vi "EventRobotResponding.vi"(9 "IA State 2":T1) -> (1 "Robot responding status":dbl[](array[numeric]), 2 "Is there a robot not responding?":bool)   [LabVIEW 2016]
uses:
  Core/AI Input.ctl
  Core/AI Robot.ctl
  Intel/Functions Enum.ctl
  Intel/AttackerStates.ctl
  Core/AI Ball.ctl
  Core/Field Size.ctl
  Core/AI Judge.ctl
  Intel/Command Enum.ctl
  Events.ctl
panel:
  in  "Array 2":bool[](array[boolean])
  in  "Array":dbl[](array[numeric])=[1.0, 1.0, 1.0, 1.0, 1.0, 1.0]
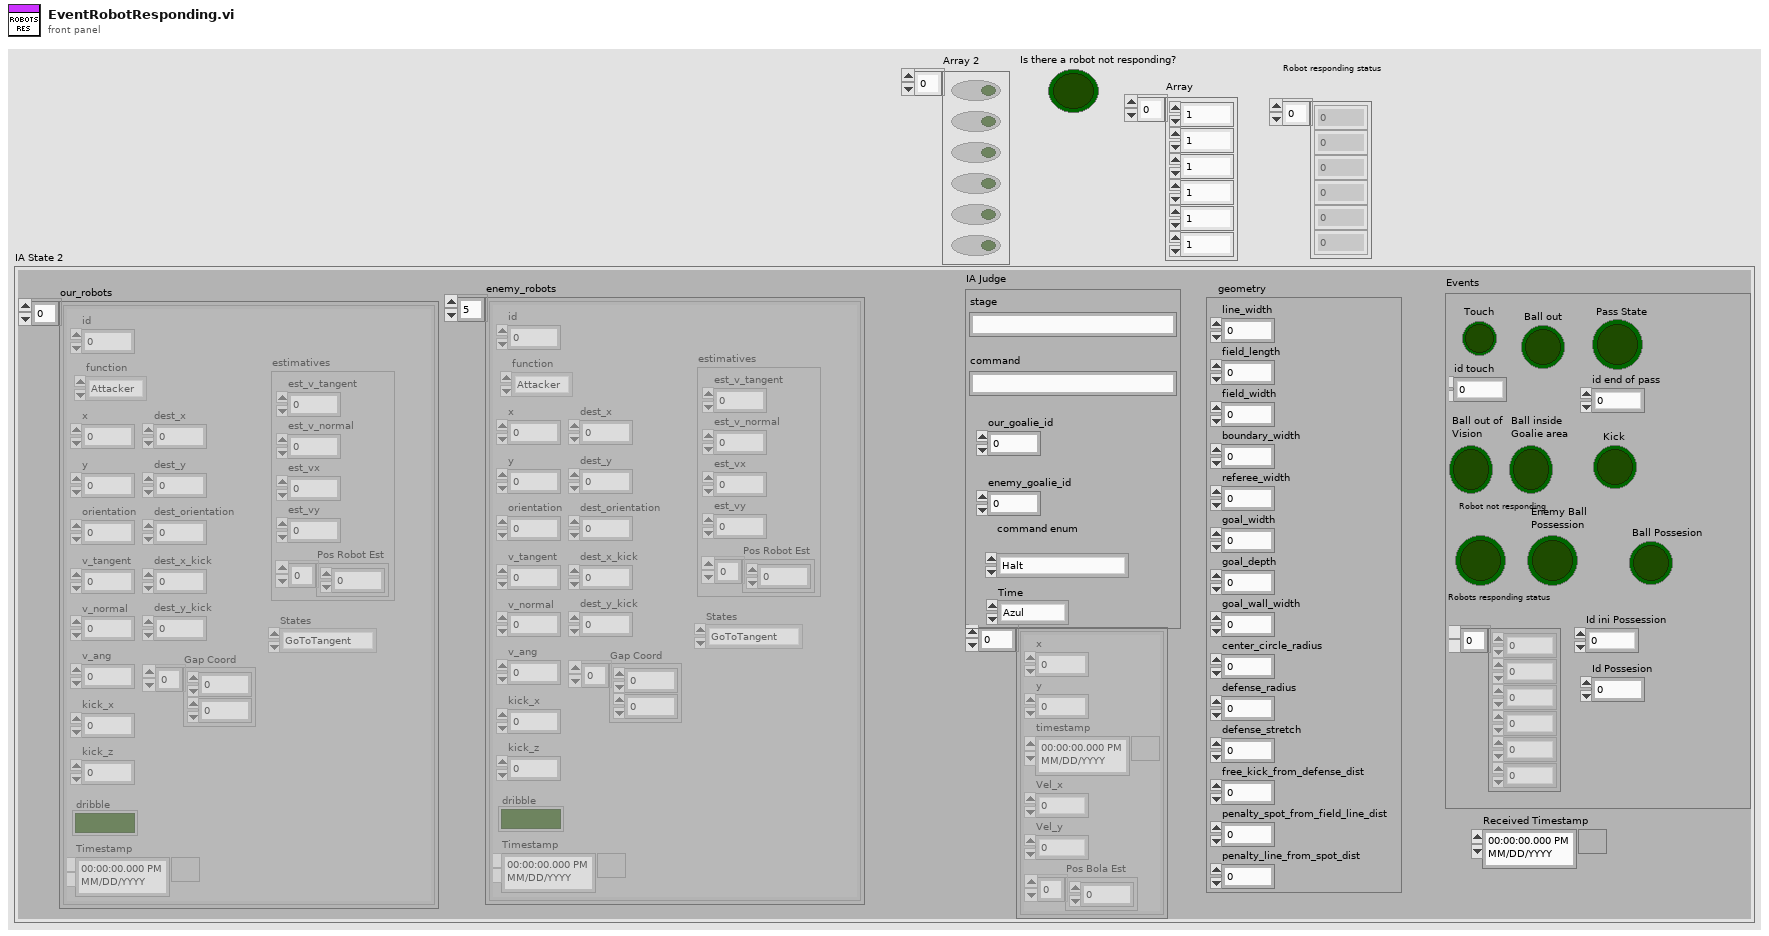
[diagram p1: front panel]
types:
  T1 = typedef "AI Input.ctl" = cluster{"our_robots":T2[], "enemy_robots":T2[], "balls":T5[], "geometry":T6, "IA Judge":T7, "Received Timestamp":timestamp, "Events":T9}
  T2 = typedef "AI Robot.ctl" = cluster{"id":u32, "function":T3, "x":dbl, "y":dbl, "orientation":dbl, "v_tangent":dbl, "v_normal":dbl, "v_ang":dbl, "kick_x":dbl, "kick_z":dbl, "dribble":bool, "Timestamp":timestamp, "dest_x":dbl, "dest_y":dbl, "dest_orientation":dbl, "estimatives":cluster{"est_v_tangent":dbl, "est_v_normal":dbl, "est_vx":dbl, "est_vy":dbl, "Pos Robot Est":dbl[]}, "dest_x_kick":dbl, "dest_y_kick":dbl, "Gap Coord":dbl[], "States":T4}
  T3 = typedef "Functions Enum.ctl" = enum16{"Attacker", "Goalie", "Defender", "Striker", "Goto 0", "Dummy", "Kicker", "ZigZag"}
  T4 = typedef "AttackerStates.ctl" = enum16{"Pass", "GoToTangent", "BallGetting", "GoToKick", ""}
  T5 = typedef "AI Ball.ctl" = cluster{"x":dbl, "y":dbl, "timestamp":timestamp, "Vel_x":dbl, "Vel_y":dbl, "Pos Bola Est":dbl[]}
  T6 = typedef "Field Size.ctl" = cluster{"line_width":u32, "field_length":u32, "field_width":u32, "boundary_width":u32, "referee_width":u32, "goal_width":u32, "goal_depth":u32, "goal_wall_width":u32, "center_circle_radius":u32, "defense_radius":u32, "defense_stretch":u32, "free_kick_from_defense_dist":u32, "penalty_spot_from_field_line_dist":u32, "penalty_line_from_spot_dist":u32}
  T7 = typedef "AI Judge.ctl" = cluster{"stage":string, "command":string, "our_goalie_id":dbl, "enemy_goalie_id":dbl, "command enum":T8, "Time":enum16{"Azul", "Amarelo"}}
  T8 = typedef "Command Enum.ctl" = enum16{"Halt", "Stop", "Force Start", "PKA Normal Start", "Prepare Kickoff Ally", "PKE Normal Start", "Prepare Kickoff Enemy", "Prepare Penalty Ally", "PPA Normal Start", "Prepare Penalty Enemy", "PPE Normal Start", "Direct Free Enemy", "Direct Free Ally", "Indirect Free Enemy", "Indirect Free Ally", "Timeout Enemy", "Timeout Ally", "Goal Enemy", "Goal Ally", "Ball Placement Enemy", "Ball Placement Ally", "Normal Half Time", "Extra Time Break", "Extra Half Time", "None", "Post Game"}
  T9 = typedef "Events.ctl" = cluster{"Touch":bool, "Ball out":bool, "id touch":dbl, "Ball out of \nVision":bool, "Ball inside \nGoalie area":bool, "Robot not responding":bool, "Robots responding status":dbl[], "Enemy Ball \nPossession":bool, "Pass State":bool, "id end of pass":dbl, "Kick":bool, "Id ini Possession":dbl, "Ball Possesion":bool, "Id Possesion":dbl}
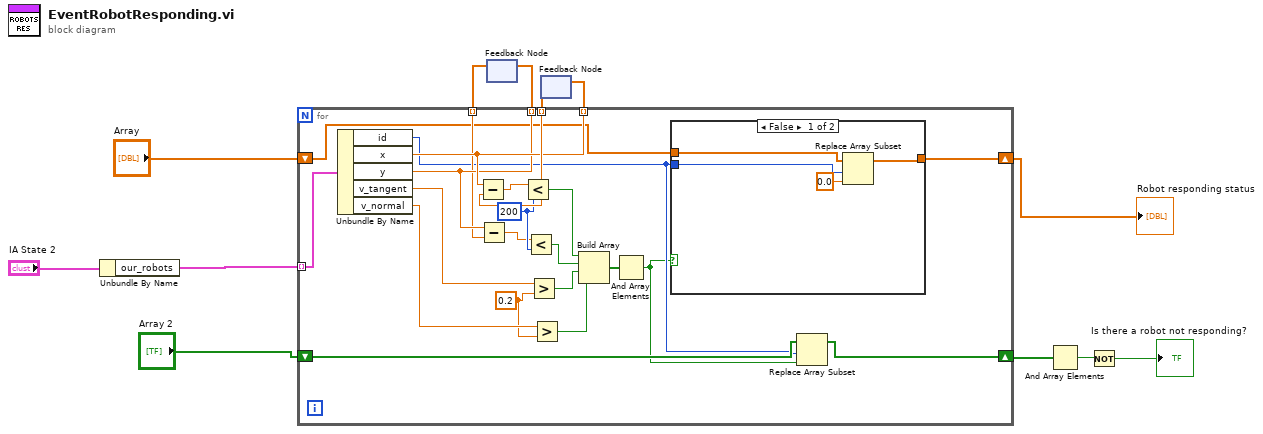
[diagram p0: block diagram]
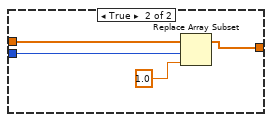
[diagram p2: hidden frame]
diagram:
  n1 = Unbundle By Name("IA State 2") -> ("our_robots"=w11:T2[])
  n2 = feedback #1() -> (w7:dbl[])  [unwired: 1 in]
  n3 = feedback #2() -> (w8:dbl[])  [unwired: 1 in]
  n4 = for {
    tunnel: w11 -> [w34] mode=indexing
    tunnel: [w32] -> w10 mode=indexing
    tunnel: [w31] -> w9 mode=indexing
    tunnel: w8 -> [w33] mode=indexing
    tunnel: w7 -> [w30] mode=indexing
    shift-right: [w18] -> w5
    shift-left: "Array" -> [w17]
    shift-right: [w13] -> w3
    shift-left: "Array 2" -> [w16]
    w24 = 0.2 ("y")
    w28 = 200
    n5 = Unbundle By Name(w34) -> ("id"=w15:u32, "x"=w32:dbl, "y"=w31:dbl, "v_tangent"=w26:dbl, "v_normal"=w25:dbl)
    n6 = Subtract(x=w32, y=w33) -> (x-y=w29:dbl)
    n7 = Subtract(x=w31, y=w30) -> (x-y=w27:dbl)
    n8 = Less?(x=w29, y=w28) -> (x < y?=w23:bool)
    n9 = Less?(x=w27, y=w28) -> (x < y?=w22:bool)
    n10 = Greater?(x=w26, y=w24) -> (0:w21:bool)
    n11 = Greater?(x=w25, y=w24) -> (0:w20:bool)
    n12 = Build Array(w23, w22, w21, w20) -> (w19:bool[])
    n13 = And Array Elements(Boolean array=w19) -> (logical AND=w14:bool)
    n14 = case shown="False" w14 {
      tunnel: [w36 w42] -> w18
      tunnel: w17 -> [w38 w41]
      tunnel: w15 -> [w37 w40]
      frame False {
        n15 = Replace Array Subset(array=w38, new element=0.0 ("new element/subarray"), index=w37) -> (w36:dbl[])
      }
      frame True {
        n16 = Replace Array Subset(array=w41, new element=1.0 ("new element/subarray"), index=w40) -> (w42:dbl[])
      }
    }
    n17 = Replace Array Subset(array=w16, new element=w14, index=w15) -> (w13:bool[])
  }
  "Robot responding status" <- w5
  n18 = feedback-in #1(w9) -> ()
  n19 = feedback-in #2(w10) -> ()
  n20 = And Array Elements(Boolean array=w3) -> (logical AND=w2:bool)
  n21 = Not(x=w2) -> (.not. x?=→"Is there a robot not responding?":bool)
